vi "testRunningView.vi"() -> ()   [LabVIEW 2015, in "ILCBTViews.lvlib"]
uses:
  ILCBTViews.lvlib
  UserEvents/UserEvents.lvclass
  UserEvents/UserEvents.lvclass/UserEvents.ctl
  Typedefs/StateSelector.ctl
  abortTestSeries.vi
  Typedefs/ILCBTTypedefs.lvlib
panel:
  in  "Abort?":bool
  out "Test Results":i32(listbox)
  out "Total Tests":i32
  out "Current Test Number":i32
  out "Currently Executing Test":string
  in  "UserEvents in":refnum<class "UserEvents.lvclass">
  # "("
  # "of"
  # ")"
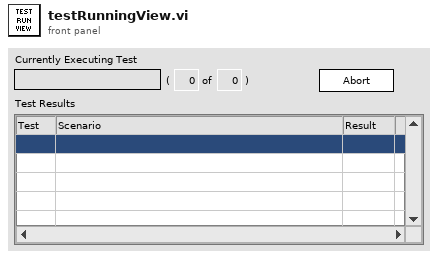
[diagram p1: front panel]
types:
  T1 = typedef "ILCBTTypedefs.lvlib/PubDataEvents.ctl" = cluster{"State":refnum<user-event>, "ErrorCode":refnum<user-event>, "OutputData":refnum<user-event>, "LogPath":refnum<user-event>, "TestScenarioCompleted":refnum<user-event>, "TestScenarioStarted":refnum<user-event>, "TestingStarted":refnum<user-event>, "StartTestScenario":refnum<user-event>}
  T2 = cluster{"Event Registration Refnum":refnum<event-registration>, "Event Registration Refnum":refnum<event-registration>, "Event Registration Refnum":refnum<event-registration>, "Event Registration Refnum":refnum<event-registration>}
  T3 = typedef "ILCBTTypedefs.lvlib/StateSelector.ctl" = enum16{"EnabledState", "FaultState", "OffState", "StandbyState", "WaitingForTestState", "ExecutingTestState"}
  T4 = typedef "ILCBTTypedefs.lvlib/TestScenarioTypes.ctl" = enum16{"+3.3VA Supply Test", "+3.3VD Supply Test", "+5VA Supply Test", "+5VD Supply Test", "Unique ID Test", "TEDS Status Test", "LIMSW1_TTL Low Test", "LIMSW1_TTL High Test", "LIMSW2_TTL Low Test", "LIMSW2_TTL High Test", "Tachometer Low Test", "Tachometer High Test", "SSR_TTL Low Test", "SSR_TTL High Test", "SM_GPI Low Test", "SM_GPI High Test", "CW Motion Without Limit Test", "CW Motion With Limit Test", "CW Motion With Both Limits Test", "CW Motion on CCW Limit Test", "CCW Motion Without Limit Test", "CCW Motion With Limit Test", "CCW Motion With Both Limits Test", "CCW Motion on CW Limit Test", "RS232-TXD Low Test", "RS232-TXD High Test", "RS232-RTS Low Test", "RS232-RTS High Test", "RS232-RXD Low Test", "RS232-RXD High Test", "RS232-CTS Low Test", "RS232-CTS High Test", "Out_SS Low Test", "Out_SS High Test", "Out_SDI Low Test", "Out_SDI High Test", "Out_SCLK Low Test", "Out_SCLK High Test", "Reset Low Test", "Reset High Test", "1 Channel ADC Test", "3 Channel ADC Test", "5 Channel ADC Test", "Vref Test", "ROT Test", "DAC1 Test", "DAC2 Test", "DAC3 Test", "DAC4 Test", "BIAS Test", "EXC1 Test", "EXC2 Test", "EXC3 Test", "EXC4 Test"}
  T5 = typedef "ILCBTTypedefs.lvlib/PassFailTest.ctl" = enum16{"Fail", "Pass", "NA"}
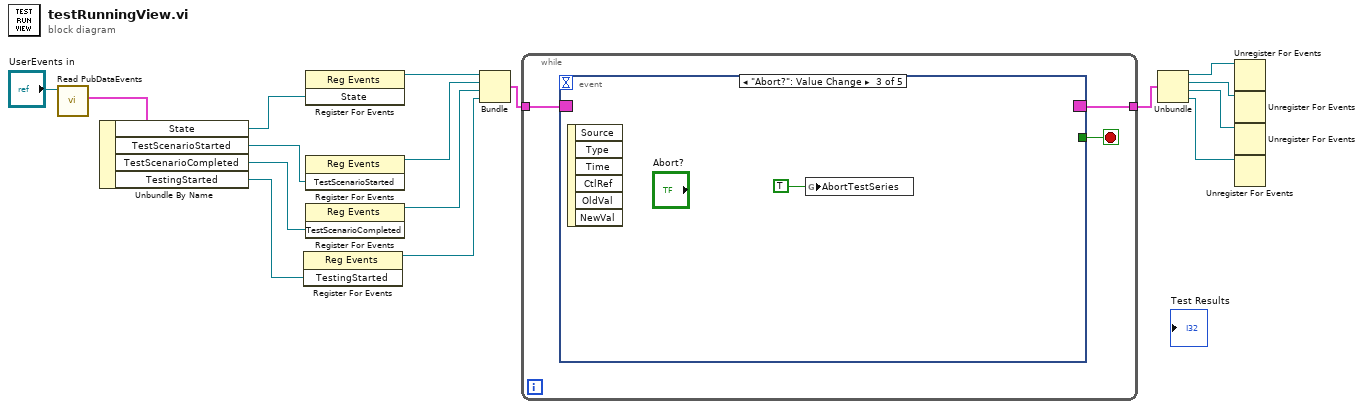
[diagram p0: block diagram]
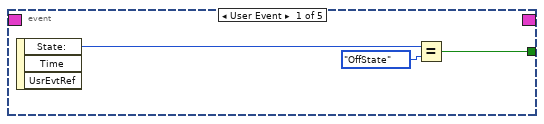
[diagram p2: hidden frame]
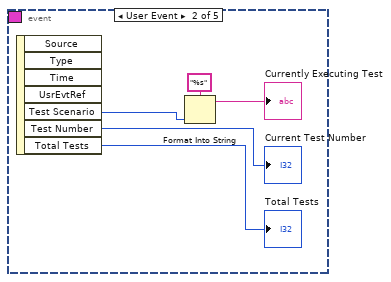
[diagram p3: hidden frame]
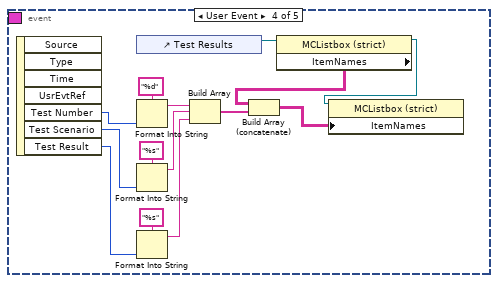
[diagram p4: hidden frame]
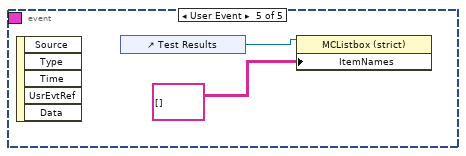
[diagram p5: hidden frame]
diagram:
  n1 = call "Read PubDataEvents.vi"("UserEvents in"="UserEvents in") -> ("PubDataEvents"=w16:T1)  [unwired: 9 in, 1 out]
  n2 = Unbundle By Name(w16) -> ("State"=w15:refnum<user-event>, "TestScenarioStarted"=w9:refnum<user-event>, "TestScenarioCompleted"=w10:refnum<user-event>, "TestingStarted"=w6:refnum<user-event>)
  n3 = register-events(w6) -> (reference out=w5:refnum<event-registration>)  [unwired: 2 in, 1 out]
  n4 = register-events(w15) -> (reference out=w14:refnum<event-registration>)  [unwired: 2 in, 1 out]
  n5 = register-events(w9) -> (reference out=w8:refnum<event-registration>)  [unwired: 2 in, 1 out]
  n6 = register-events(w10) -> (reference out=w7:refnum<event-registration>)  [unwired: 2 in, 1 out]
  n7 = Bundle("Event Registration Refnum"=w14, "Event Registration Refnum"=w8, "Event Registration Refnum"=w7, "Event Registration Refnum"=w5) -> (w12:T2)  [unwired: 1 in]
  n8 = while {
    tunnel: w12 -> [w19]
    tunnel: [w17] -> w11
    stop <- w18 stop-if-true
    n9 = event shown="[2] \"Abort?\": Value Change" {
      selector: w19 -> [_ _ _ _ _]
      dyn-events: [_ _ _ _ _] -> w17
      timeout: _ -> [_ _ _ _ _]
      tunnel: [w21 _ _ _ _] -> w18
      event User Event {
        n10 = event-data() -> ("State:"=w20:T3)  [unwired: 1 in, 2 out]
        n11 = Equal?(x=w20, y=StateSelector."OffState" ("State:")) -> (x = y?=w21:bool)
      }
      event User Event {
        n12 = event-data() -> ("Test Scenario"=w25:T4, "Test Number"=→"Current Test Number":i32, "Total Tests"=→"Total Tests":i32)  [unwired: 1 in, 4 out]
        n13 = Format Into String(format string="%s", w25) -> (resulting string=→"Currently Executing Test":string)  [unwired: 2 in, 1 out]
      }
      event "Abort?": Value Change {
        n14 = event-data() -> ()  [unwired: 1 in, 6 out]
        n15 = global write "abortTestSeries.vi" "AbortTestSeries"(TRUE ("AbortTestSeries")) -> ()
      }
      event User Event {
        n16 = event-data() -> ("Test Number"=w35:i32, "Test Scenario"=w36:T4, "Test Result"=w37:T5)  [unwired: 1 in, 4 out]
        n17 = control-ref of="Test Results"() -> (w42:refnum<vi>)
        n18 = Format Into String(format string="%d", w35) -> (resulting string=w34:string)  [unwired: 2 in, 1 out]
        n19 = Format Into String(format string="%s", w36) -> (resulting string=w33:string)  [unwired: 2 in, 1 out]
        n20 = Format Into String(format string="%s", w37) -> (resulting string=w32:string)  [unwired: 2 in, 1 out]
        n21 = Build Array(w34, w33, w32) -> (w31:string[])
        n22 = property class="MCListbox (strict)"(reference=w42) -> (reference out=w30:refnum<vi>, "ItemNames"=w41:string[][])  [unwired: 1 in, 1 out]
        n23 = Build Array (concatenate)(w41, w31) -> (w29:string[][])
        n24 = property class="MCListbox (strict)"(reference=w30, "ItemNames"=w29) -> ()  [unwired: 1 in, 2 out]
      }
      event User Event {
        n25 = event-data() -> ()  [unwired: 1 in, 5 out]
        n26 = control-ref of="Test Results"() -> (w44:refnum<vi>)
        n27 = property class="MCListbox (strict)"(reference=w44, "ItemNames"=string[][] []) -> ()  [unwired: 1 in, 2 out]
      }
    }
  }
  n28 = Unbundle(w11) -> ("Event Registration Refnum"=w4:refnum<event-registration>, "Event Registration Refnum"=w3:refnum<event-registration>, "Event Registration Refnum"=w2:refnum<event-registration>, "Event Registration Refnum"=w1:refnum<event-registration>)
  n29 = Unregister For Events(event registration refnum=w4) -> ()  [unwired: 1 in, 1 out]
  n30 = Unregister For Events(event registration refnum=w3) -> ()  [unwired: 1 in, 1 out]
  n31 = Unregister For Events(event registration refnum=w2) -> ()  [unwired: 1 in, 1 out]
  n32 = Unregister For Events(event registration refnum=w1) -> ()  [unwired: 1 in, 1 out]
